vi "ArmAutoTargetingExtension.vi"() -> (0 "Arm Extension (in)":dbl)   [LabVIEW 2020]
doc: "Determines how much extra the arm should extend to compensate for its current pose."
uses:
  GlobalDrivebase.vi
  GlobalPoseAndTargeting.vi
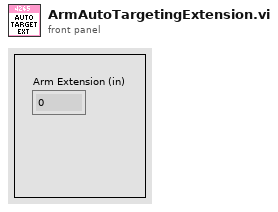
[diagram p1: front panel]
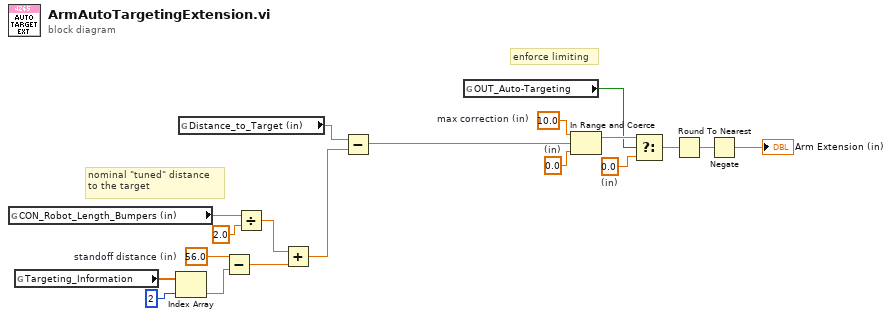
[diagram p0: block diagram]
diagram:
  w5 = 10.0  # max correction (in)
  w11 = 56.0  # standoff distance (in)
  w8 = 0.0  # (in)
  w4 = 0.0  # (in)
  # "enforce limiting"
  # "nominal \"tuned\" distance\nto the target"
  n1 = global read "GlobalDrivebase.vi" "CON_Robot_Length_Bumpers (in)"() -> (w15:dbl)
  n2 = global read "GlobalPoseAndTargeting.vi" "Targeting_Information"() -> (w9:dbl[])
  n3 = Index Array(array=w9, index=2) -> (element=w12:dbl)
  n4 = global read "GlobalPoseAndTargeting.vi" "Distance_to_Target (in)"() -> (w13:dbl)
  n5 = Subtract(x=w11, y=w12) -> (x-y=w14:dbl)
  n6 = Divide(x=w15, y=2.0) -> (x/y=w17:dbl)
  n7 = Add(x=w17, y=w14) -> (x+y=w18:dbl)
  n8 = Subtract(x=w13, y=w18) -> (x-y=w19:dbl)
  n9 = global read "GlobalDrivebase.vi" "OUT_Auto-Targeting"() -> (w6:bool)
  n10 = In Range and Coerce(upper limit=w5, x=w19, lower limit=w4) -> (coerced(x)=w7:dbl)  [unwired: 1 out]
  n11 = Select(t=w7, s=w6, f=w8) -> (s? t:f=w2:dbl)
  n12 = Round To Nearest(number=w2) -> (nearest integer value=w1:dbl)
  n13 = Negate(x=w1) -> (-x=→"Arm Extension (in)":dbl)
